vi "Read Trace Buffer.vi"(8 "error in (no error)":errorcluster, 10 "Channel (0: Channel 1)":i32(ring) items=["Channel 1", "Channel 2"], 11 "VISA resource name":refnum<visa-resource-name>) -> (0 "error out":errorcluster, 2 "Trace Buffer Data":dbl[](array[numeric]), 3 "VISA resource name out":refnum<visa-resource-name>)   [LabVIEW 2023, in "Agilent B2900 Series.lvlib"]
doc: "Reads the data in the trace buffer."
uses:
  Agilent B2900 Series.lvlib
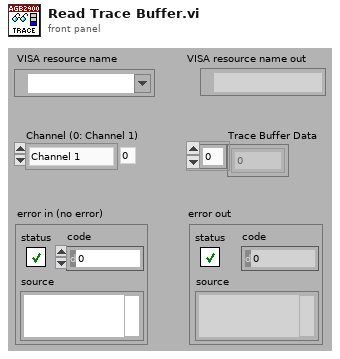
[diagram p1: front panel]
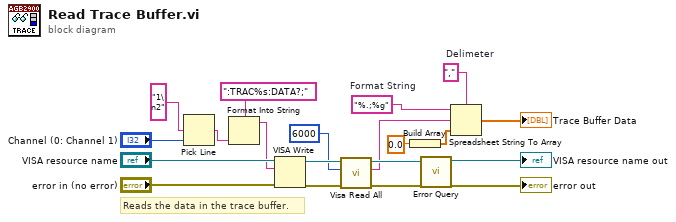
[diagram p0: block diagram]
diagram:
  w13 = ","  # Delimeter
  w16 = "%.;%g"  # Format String
  # "Reads the data in the trace buffer."
  n1 = Pick Line(multi-line string="1\n2" ("string (\"\")"), line index="Channel (0: Channel 1)") -> (output string=w7:string)  [unwired: 1 in]
  n2 = Format Into String(format string=":TRAC%s:DATA?;", w7) -> (resulting string=w10:string)  [unwired: 2 in, 1 out]
  n3 = VISA Write(VISA resource name="VISA resource name", write buffer=w10, error in (no error)="error in (no error)") -> (VISA resource name out=w3:refnum<visa-resource-name>, error out=w4:errorcluster)  [unwired: 1 out]
  n4 = call "Visa Read All.vi"("error in (no error)"=w4, "Byte Count Each Loop (6000)"=u32 6000 ("byte count"), "VISA resource name"=w3) -> ("error out"=w5:errorcluster, "Read Buffer"=w1:string, "VISA resource name out"=w6:refnum<visa-resource-name>)  [unwired: 6 in]
  n5 = Build Array(0.0) -> (w15:dbl[])
  n6 = call "Error Query.vi"("error in (no error)"=w5, "VISA resource name"=w6) -> ("error out"=→"error out":errorcluster, "VISA resource name out"=→"VISA resource name out":refnum<visa-resource-name>)  [unwired: 6 in, 2 out]
  n7 = Spreadsheet String To Array(delimiter (Tab)=w13, format string=w16, spreadsheet string=w1, array type (2D Dbl)=w15) -> (array=→"Trace Buffer Data":dbl[])
